vi "WRP Get Detector Info.vi"(8 "error in (no error)":errorcluster) -> (0 "error out":errorcluster, 2 "function return":i32, 3 "value":T1)   [LabVIEW 2018, in "SesWrapper.lvlib"]
doc: "int STDCALL WRP_GetDetectorInfo(DetectorInfo *value);"
uses:
  SesWrapper.lvlib
  build/Debug/SESWrapper.dll
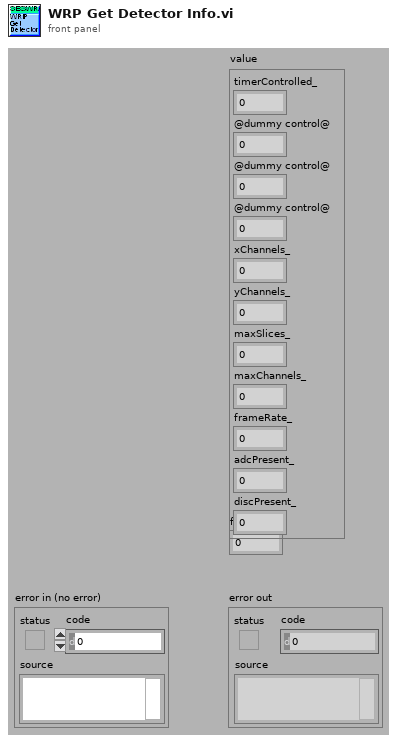
[diagram p1: front panel]
types:
  T1 = cluster{"timerControlled_":u8, "@dummy control@":i8, "@dummy control@":i8, "@dummy control@":i8, "xChannels_":i32, "yChannels_":i32, "maxSlices_":i32, "maxChannels_":i32, "frameRate_":i32, "adcPresent_":u8, "discPresent_":u8}
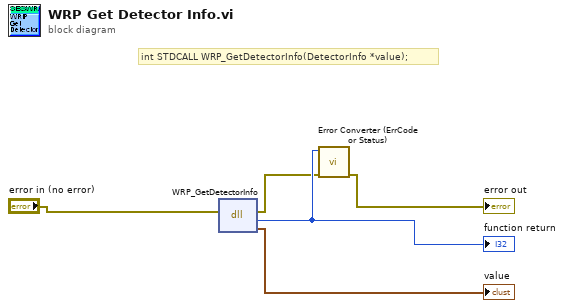
[diagram p0: block diagram]
diagram:
  # "int STDCALL WRP_GetDetectorInfo(DetectorInfo *value);"
  n1 = dll-call lib="C:/Development/svn/seswrapper-lib/build/Debug/SESWrapper.*" fn="WRP_GetDetectorInfo"(error in="error in (no error)") -> (error out=w2:errorcluster, w5:i32, "value"=→"value":T1)  [unwired: 3 in, 1 out]
  "function return" <- w5
  n2 = call "Error Converter (ErrCode or Status).vi"("error in (no error)"=w2, "error code"=w5) -> ("error out"=→"error out":errorcluster)  [unwired: 9 in]
